vi "Periodic Tasks.vi"(8 "error in":errorcluster) -> ()   [LabVIEW 2014]
doc: "This VI runs in parallel to other tasks. It can contain as many user-defined periodic loops as you need. These can carry out PID or other sorts of timed response."
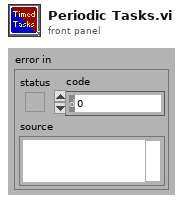
[diagram p1: front panel]
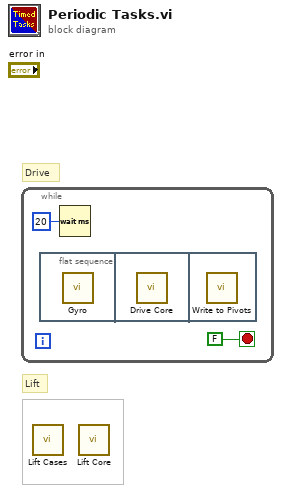
[diagram p0: block diagram]
diagram:
  # "Drive"
  # "Lift"
  n1 = while {
    stop <- FALSE stop-if-true
    n2 = flat-sequence {
      frame #0 {
        n3 = call "Gyro.vi"() -> ()  [unwired: 12 in]
      }
      frame #1 {
        n4 = call "Drive Core.vi"() -> ()  [unwired: 12 in]
      }
      frame #2 {
        n5 = call "Write to Pivots.vi"() -> ()  [unwired: 12 in]
      }
    }
    n6 = Wait (ms)(milliseconds to wait=u32 20) -> ()  [unwired: 1 out]
  }
  n7 = call "Lift Cases.vi"() -> ()  [unwired: 12 in]
  n8 = call "Lift Core.vi"() -> ()  [unwired: 12 in]
